vi "VI Stoermeldeverwaltung.vi"(8 "error in (no error)":errorcluster caption="Fehler (Eingang)") -> (0 "error out":errorcluster caption="Fehler (Ausgang)")   [LabVIEW 2020, in "Stoerungen.lvlib"]
uses:
  Stoerungen/Stoerungen.lvlib
  Stoerungen/FGV Stoerung aufnehmen Aktion.ctl
  Seiten/Erweiterte Konfig/FGV PID Aktionen.ctl
  Funktionstasten/Funktionstasten-Aktion.ctl
  Funktionstasten/Zustaende.ctl
  Funktionstasten/Funktionstasten.lvlib
  Seiten/Erweiterte Konfig/Erweiterte Konfig.lvlib
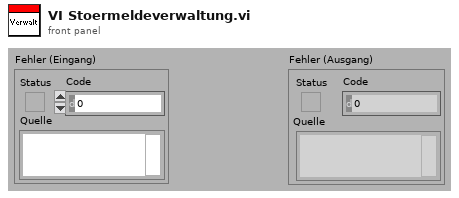
[diagram p1: front panel]
types:
  T1 = typedef "Funktionstasten.lvlib/Funktionstasten-Aktion.ctl" = enum16{"Initialisieren", "Zustand setzen", "Taste gedrückt", "Fehler speichern", "Lesen", "Manuell", "Remote", "Bitparallel", "Samplepoint", "Zeit Prüfen", "reset Umschalten"}
  T2 = typedef "Erweiterte Konfig.lvlib/FGV PID Aktionen.ctl" = enum16{"Lesen", "Schreiben PID", "Schreiben Sonstige", "Dichtheitstest", "Aktionen Dicht.", "Parameter Sensor"}
  T3 = typedef "Stoerungen.lvlib/FGV Stoerung aufnehmen Aktion.ctl" = enum16{"Initialisieren", "Schreiben", "Lesen", "Quittieren", "quit. löschen"}
  T4 = typedef "Funktionstasten.lvlib/Zustaende.ctl" = enum16{"Standby", "Pause", "Eco", "Messen", "Kalibrieren", "Spülen Filter", "Spülen Leitung", "Umgebungsluft", "0-Gas", "Cal-Gas", "CG zu PNS", "-------------", "Init 1", "Init 2", "Init 3", "Init 4", "Messen vorbereiten", "Messen durchführen", "Exit"}
  T5 = typedef "Erweiterte Konfig.lvlib/Sonstige Parameter.ctl" = cluster{"Lüfter langsam":sgl, "Lüfter schnell":sgl, "FT-IR Kühlung Soll":sgl, "FT-IR Kühlung Max":sgl, "Überwachung":T6, "Befüllung aktiv":T7, "Stickstoff Befüllzeit":sgl, "Befüllintervall":sgl, "Kalibrierwert FT-IR":sgl, "Offset Ausgang":sgl, "Offset FT-IR":sgl, "Offset Druck FT-IR":sgl, "Dichtheitstest Zeit":sgl, "Dichtheitstest Abfall":sgl, "Dichtheitstest Umfang":T8, "Offset Umgebung":sgl, "Max Taupunkt":sgl, "Pumpendrehzahl":sgl, "ext. Befüllung":T7, "Ext. Stickstoff Befüllzeit":sgl}
  T6 = typedef "Auswahlfeld.ctl" = u16
  T7 = typedef "LogKonfig.lvlib/Auswahlfeld aktiviert-deaktiviert.ctl" = u16
  T8 = typedef "Erweiterte Konfig.lvlib/Dichtheitstest Umfang.ctl" = u16
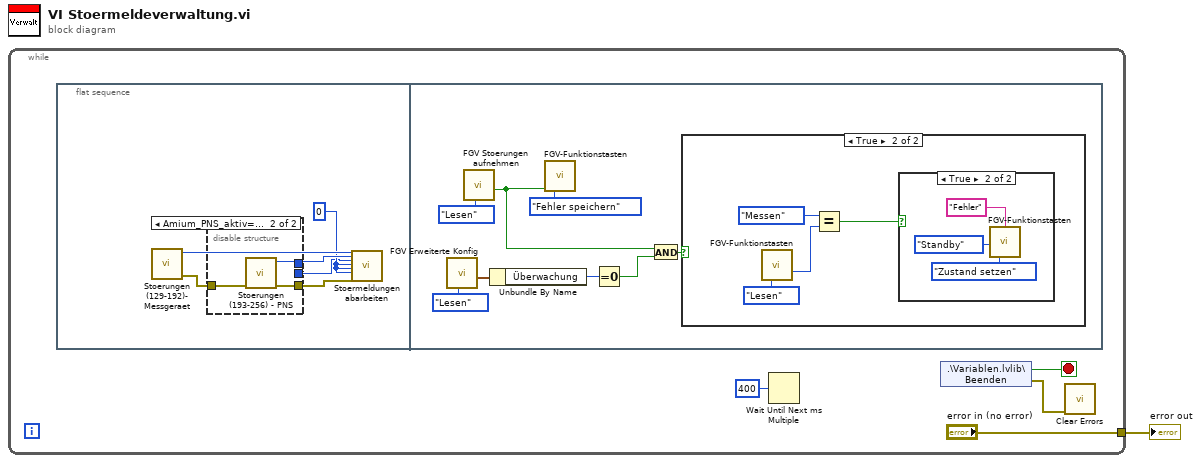
[diagram p0: block diagram]
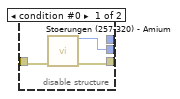
[diagram p2: hidden frame]
diagram:
  n1 = while {
    tunnel: ["error in (no error)"] -> w1
    stop <- w4 stop-if-true
    n2 = flat-sequence {
      frame #0 {
        w7 = u64 0 ("Störungen 257-320")
        n3 = call "Stoerungen (129-192)- Messgeraet.vi"() -> ("Fehler (Ausgang)"=w10:errorcluster, "Störungen 129-192"=w11:u64)  [unwired: 10 in]
        n4 = disable-structure shown="Amium_PNS_aktiv==FALSE" {
          disable-tunnel: w10 -> [w14 w17]
          disable-tunnel: [_ w16] -> w9
          disable-tunnel: [w13 w15] -> w8
          disable-tunnel: [w12 _] -> w6
          frame condition #0 {
            n5 = call "Stoerungen (257-320) - Amium.vi"("Fehler (Eingang)"=w14) -> ("Fehler (Ausgang)"=w13:errorcluster, "Störungen 257-320"=w12:u64)  [unwired: 9 in]
          }
          frame condition #1 (active) {
            n6 = call "Stoerungen (193-256) - PNS.vi"("Fehler (Eingang)"=w17) -> ("Fehler (Ausgang)"=w15:errorcluster, "Störungen 193-256"=w16:u64)  [unwired: 9 in]
          }
        }
        n7 = call "Stoermeldungen abarbeiten.vi"("Störungen 129-192"=w11, "Störungen 193-256"=w9, "Störungen 257-320"=w6, "Störungen 321-384"=w7, "Störungen 385-448"=w7, "Störungen 449-512"=w7, "Fehler (Eingang)"=w8) -> ()  [unwired: 20 in, 1 out]
      }
      frame #1 {
        n8 = call "FGV Erweiterte Konfig.vi"("Aktion"=FGV_PID_Aktionen."Lesen") -> ("Sonstige"=w25:T5)  [unwired: 6 in, 4 out]
        n9 = call "FGV Stoerungen aufnehmen.vi"("FGV Störung aufnehmen Aktion"=FGV_Stoerung_aufnehmen_Aktion."Lesen") -> ("abschalten"=w18:bool)  [unwired: 7 in, 3 out]
        n10 = Unbundle By Name(w25) -> ("Überwachung"=w20:T6)
        n11 = call "FGV-Funktionstasten.vi"("Fehler (FALSE)"=w18, "Aktion"=Funktionstasten-Aktion."Fehler speichern") -> ()  [unwired: 6 in, 8 out]
        n12 = Equal To 0?(x=w20) -> (x = 0?=w21:bool)
        n13 = And(x=w18, y=w21) -> (x .and. y?=w23:bool)
        n14 = case shown="True" w23 {
          frame False {
          }
          frame True {
            n15 = call "FGV-Funktionstasten.vi"("Aktion"=Funktionstasten-Aktion."Lesen") -> ("ausgewählte Funktion"=w28:T4)  [unwired: 7 in, 7 out]
            n16 = Equal?(x=Zustaende."Messen", y=w28) -> (x = y?=w26:bool)
            n17 = case shown="True" w26 {
              frame False {
              }
              frame True {
                n18 = call "FGV-Funktionstasten.vi"("Herkunft"="Fehler", "Zustand"=Zustaende."Standby", "Aktion"=Funktionstasten-Aktion."Zustand setzen") -> ()  [unwired: 5 in, 8 out]
              }
            }
          }
        }
      }
    }
    n19 = Wait Until Next ms Multiple(millisecond multiple=u32 400 ("Vielfache von ms")) -> ()  [unwired: 1 out]
    n20 = shared-variable ".\\Variablen.lvlib\\Beenden"() -> (w4:bool, error out=w2:errorcluster)  [unwired: 1 out]
    n21 = call <vilib>:"Clear Errors.vi"("error in (no error)"=w2) -> ()  [unwired: 5 in, 2 out]
  }
  "error out" <- w1
